vi "XYZStage-Request movement stop.vi"(9 "Pos ctrl window queue":refnum<queue>) -> ()   [LabVIEW 2013]
uses:
  User Interface/Windows/Position control window/Typedefs/Pos Ctrl queue data cluster.ctl
  User Interface/Windows/Position control window/Typedefs/Pos Ctrl States.ctl
  Typedefs/XYZ stage states.ctl
  Typedefs/XYZ stage data.ctl
  Typedefs/XYZ channel ring.ctl
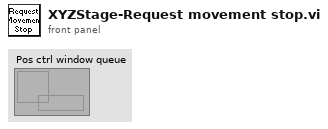
[diagram p1: front panel]
types:
  T1 = typedef "XYZ stage data.ctl" = cluster{"Command":T2, "Channel":T3, "X":sgl, "Y":sgl, "Z":sgl, "Speed":i32, "Zero":bool, "Use acknowledgement?":bool}
  T2 = typedef "XYZ stage states.ctl" = enum16{"Dequeue", "Initialize", "Read Position", "Read Speed Setting", "Move", "Set Max Speed", "Reset Axis", "Stop all movement"}
  T3 = typedef "XYZ channel ring.ctl" = string
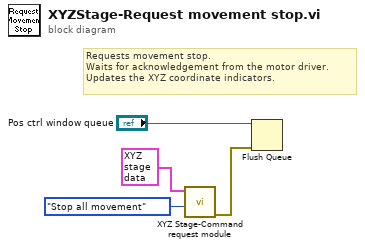
[diagram p0: block diagram]
diagram:
  # "Requests movement stop.\nWaits for acknowledgement from the motor driver.\nUpdates the XYZ coordinate indicators."
  n1 = call "XYZ Stage-Command request module.vi"("Command"=XYZ_stage_states."Stop all movement", "XYZ Stage data to queue"=T1 {"Command"=enum."Initialize", "Channel"="Z", "X"=0.0, "Y"=0.0, "Z"=0.0, "Speed"=0, "Zero"=FALSE, "Use acknowledgement?"=FALSE}) -> ("error out"=w1:errorcluster)  [unwired: 5 in, 4 out]
  n2 = Flush Queue(queue="Pos ctrl window queue", error in (no error)=w1) -> ()  [unwired: 3 out]
